vi "Generate Trace.vi"(10 "Trace String":string, 11 "AF Trace Queue in":refnum<class "AF Trace Queue.lvclass">) -> (3 "AF Trace Queue out":refnum<class "AF Trace Queue.lvclass">)   [LabVIEW 2020, in "AF Trace Queue.lvclass"]
uses:
  AF Trace Queue.lvclass
  AF Trace Queue.lvclass/AF Trace Queue.ctl
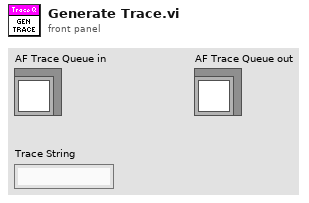
[diagram p1: front panel]
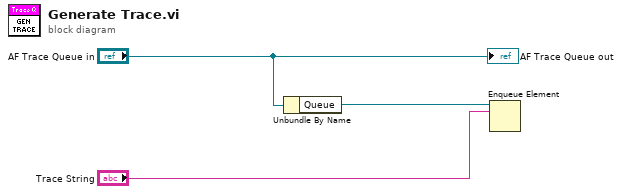
[diagram p0: block diagram]
diagram:
  n1 = Unbundle By Name("AF Trace Queue in") -> ("Queue"=w2:refnum<queue>)
  n2 = Enqueue Element(queue=w2, element="Trace String") -> ()  [unwired: 2 in, 3 out]
  "AF Trace Queue out" <- "AF Trace Queue in"
